vi "Main Page.vi"(8 "error in (no error)":errorcluster, 11 "Node Ptr":T2 format="%.0x") -> (0 "error out":errorcluster)   [LabVIEW 2016, in "DCM System Explorer.lvlib"]
uses:
  DCM System Explorer.lvlib
  <vilib>/NI Veristand/Custom Device API/Custom Device Item Ref.ctl
  Types/Bitfile Selection.ctl
  System.Windows.Forms
  <vilib>/NI Veristand/Custom Device API/Dependent File Optional Info.ctl
  <vilib>/Powertrain Controls/Device Drivers/DCM/Rev0/RT/DCM - RT.lvclass/DCM - RT.ctl
  <vilib>/Powertrain Controls/Device Drivers/DCM/Rev0/RT/Read System.vi
  <vilib>/Powertrain Controls/Device Drivers/DCM/Rev0/RT/Read PB.vi
  Shared/DCM Properties.vi
  <vilib>/NI Veristand/Custom Device API/Set Item Property (Boolean).vi
  Shared/DCM Constants and GUIDs.vi
  <vilib>/NI Veristand/Custom Device API/Get Item Property (String).vi
  <vilib>/NI Veristand/Custom Device API/Get Item Property (I32).vi
  <vilib>/NI Veristand/Custom Device API/Get Item Property (Dependent File).vi
  <vilib>/NI Veristand/Custom Device API/Get Item Property (U16).vi
  SubVIs/Custom Device Ref.vi
  <vilib>/NI Veristand/Custom Device API/Set Item Property (String).vi
  <vilib>/NI Veristand/Custom Device API/Set Item Property (U16).vi
  <vilib>/NI Veristand/Custom Device API/Set Item Property (I32).vi
  <vilib>/NI Veristand/Custom Device API/Set Item Property (Dependent File).vi
  <vilib>/NI Veristand/Custom Device API/Set Item Property (Path).vi
  <vilib>/FPGAPlugInAG/sbRIO-9651/niLvFpga_Open_sbRIO-9651.vi
  <vilib>/rvi/interface/common/dynamic/niFpgaDynamicAddResources.vi
  <vilib>/rvi/interface/nirviOpenFPGA/nirviOpenFPGA.xnode
  <vilib>/Powertrain Controls/Device Drivers/DCM/Top Level/FPGA Bitfiles/DCM - FPGA - Calibration.lvbitx
  <vilib>/NI VeriStand/Custom Device API/Custom Device API.lvlib
  DCM Shared.lvlib
  <vilib>/Powertrain Controls/Device Drivers/DCM/Rev0/RT/DCM - RT.lvclass
panel:
  in  "Password":string
  in  "Username":string
  out "Status":string
  in  "Clear":bool
  in  "Discover":bool
  in  "Header 4":cluster{"Section Name":string}={"Section Name"="Timed Loop Setup"}
  in  "Device Name":string
  in  "CPU-Sys":i32=-2 caption="CPU"
  in  "Rate-Sys":i32=1 caption="Rate decimation" min=1
  in  "Priority-Sys":enum16{"Low", "Medium", "High"}(ring)=enum."Medium" caption="Execution priority"
  in  "CPU-Cmd":i32=-2 caption="CPU"
  in  "Rate-Cmd":i32=1 caption="Rate decimation" min=1
  in  "Priority-Cmd":enum16{"Low", "Medium", "High"}(ring)=enum."Medium" caption="Execution priority"
  in  "Header 3":cluster{"Section Name":string}={"Section Name"="DCM Model & Bitfile Initialization"}
  in  "Header 2":cluster{"Section Name":string}={"Section Name"="FPGA Target Setup"}
  in  "FPGA Resource":string="RIO0"
  in  "IP Address":string
  in  "FPGA Location":enum16{"Local", "Remote"}(ring)
  out "RT File Path":string caption="RT File Path - FPGA Bitfile"
  out "Local File Path":path caption="Local File Path - FPGA Bitfile"
  out "DCM Model":T1
  out "Device Address":string="RIO0"
  out "CD Version":string caption="Custom Device Version"
  in  "Header":cluster{"Section Name":string}={"Section Name"="Real-Time Target Setup"}
  # "Command Loop"
  # "(-2: automatic)"
  # "System Loop"
  # "(-2: automatic)"
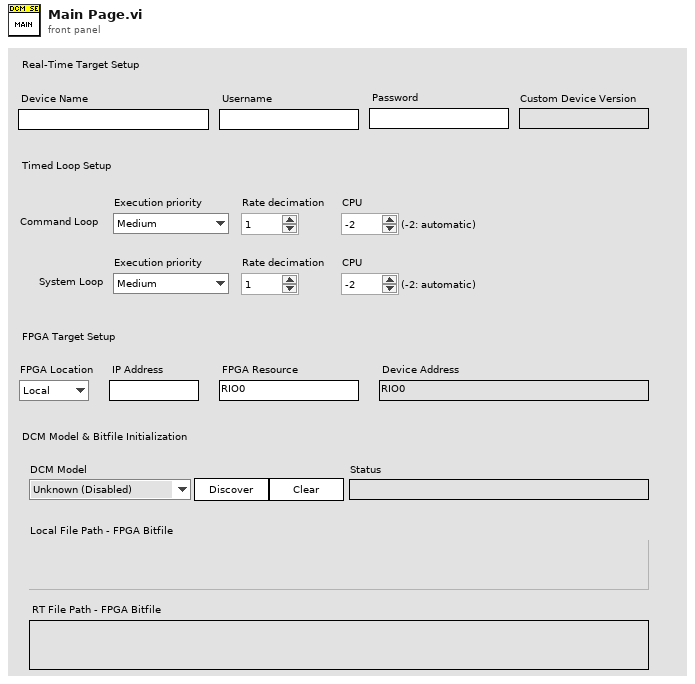
[diagram p1: front panel]
types:
  T1 = typedef "DCM System Explorer.lvlib/Bitfile Selection.ctl" = enum16{"Unknown (Disabled)", "DCM-2301", "DCM-2302", "DCM-2316", "DCM-2317"}
  T2 = typedef "Custom Device API.lvlib/Custom Device Item Ref.ctl" = u64
  T3 = enum8{"Enabled", "Disabled", "Disabled and Grayed Out"}
  T4 = typedef "Custom Device API.lvlib/Dependent File Optional Info.ctl" = cluster{"Version":string, "RTDestination":path, "ForceDownload":bool, "SupportedTarget":string, "MD5":string}
  T5 = typedef "Custom Device API.lvlib/Custom Device Item Info.ctl" = cluster{"Name":string, "Is Channel":bool, "GUID":string, "Is Waveform":bool}
  T6 = typedef "Custom Device API.lvlib/Custom Device Commands.ctl" = enum16{"Default", "Item renamed", "Shutdown", "Dynamic button pressed"}
  T7 = typedef "nirio_resource_slv.ctl" = tag
  T8 = typedef "DCM - RT.lvclass/System.ctl" = cluster{"Model":u16, "Rev Major":u8, "Rev Minor":u8, "Serial Number":u32}
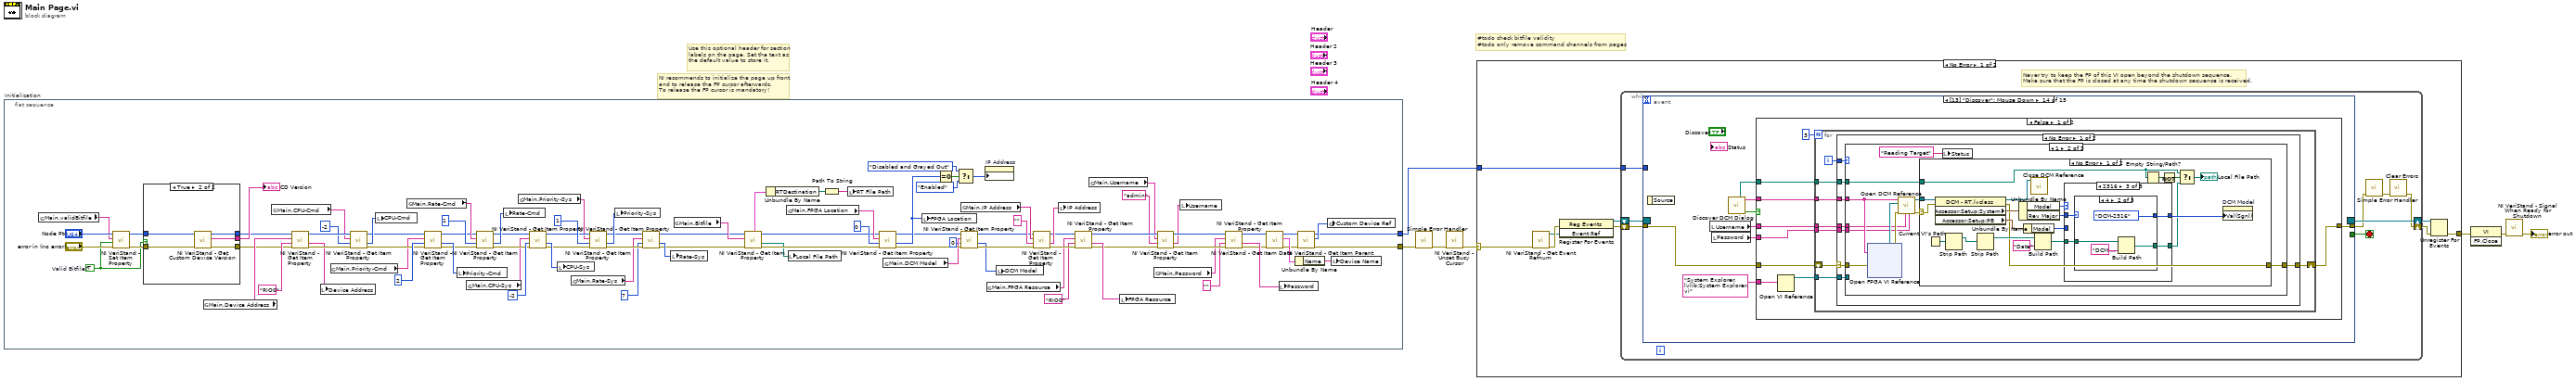
[diagram p0: block diagram]
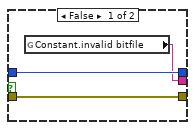
[diagram p2: hidden frame]
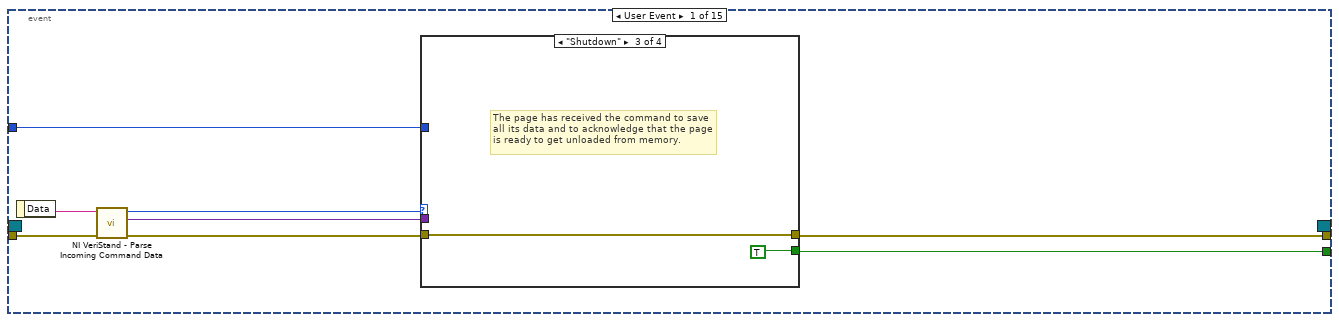
[diagram p3: hidden frame]
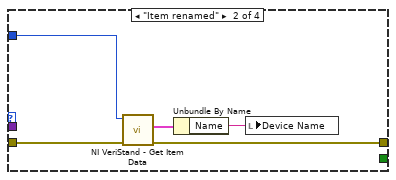
[diagram p5: hidden frame]
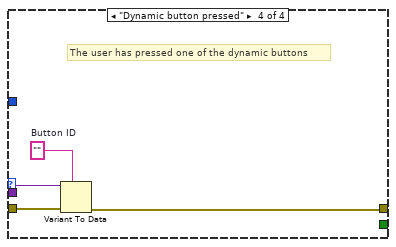
[diagram p6: hidden frame]
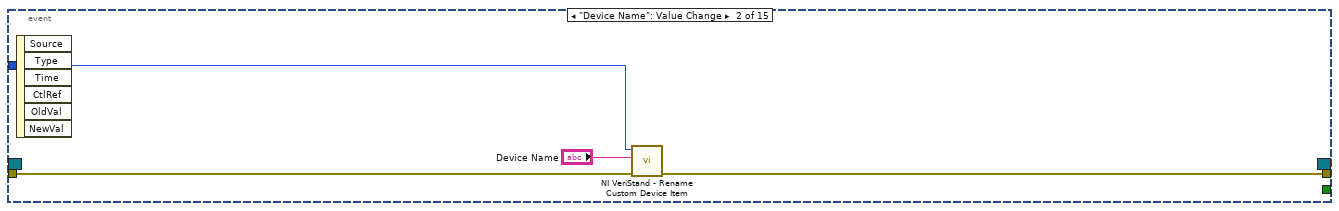
[diagram p7: hidden frame]
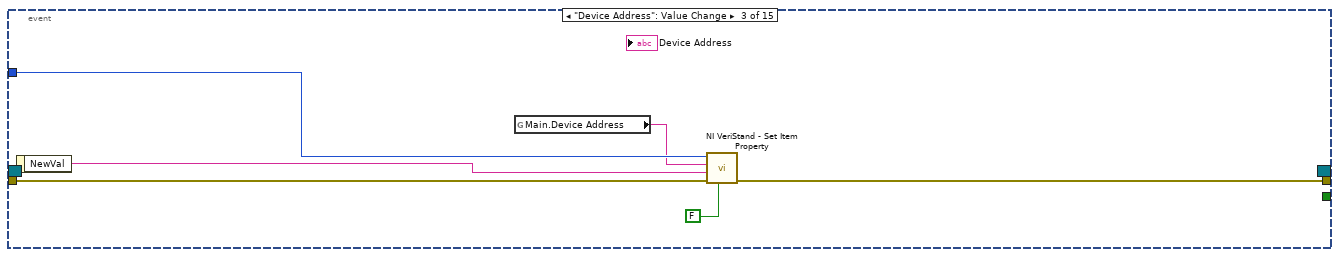
[diagram p8: hidden frame]
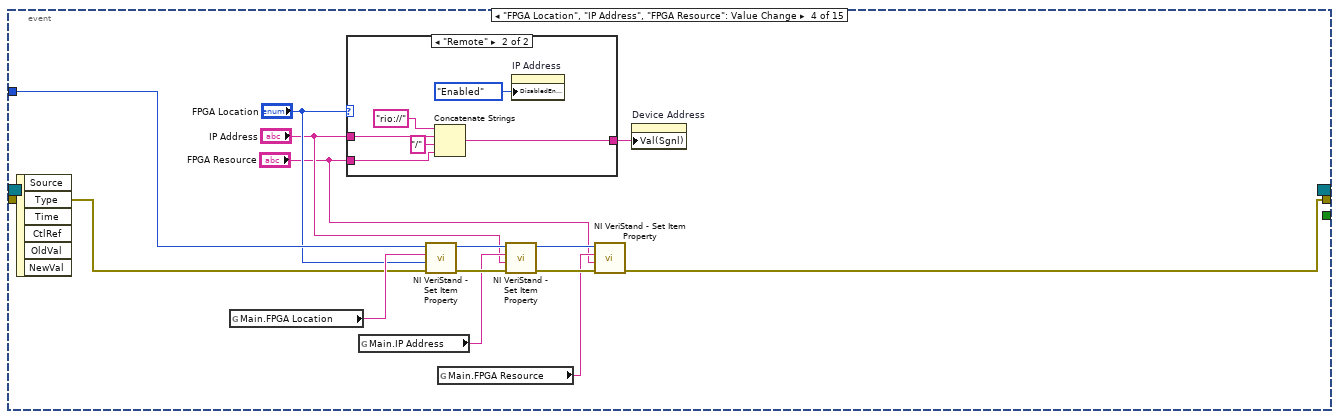
[diagram p9: hidden frame]
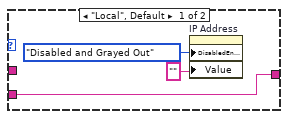
[diagram p10: hidden frame]
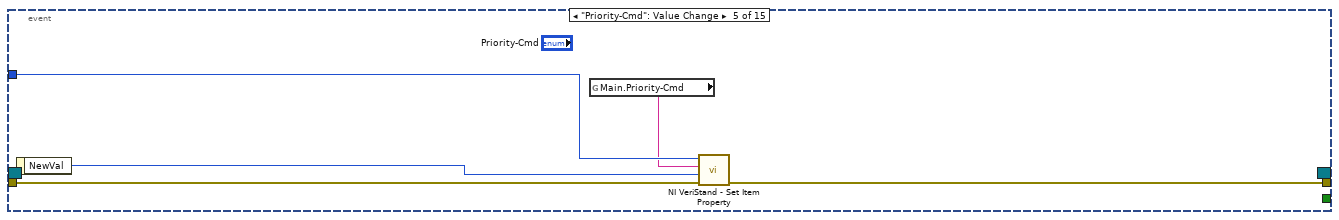
[diagram p11: hidden frame]
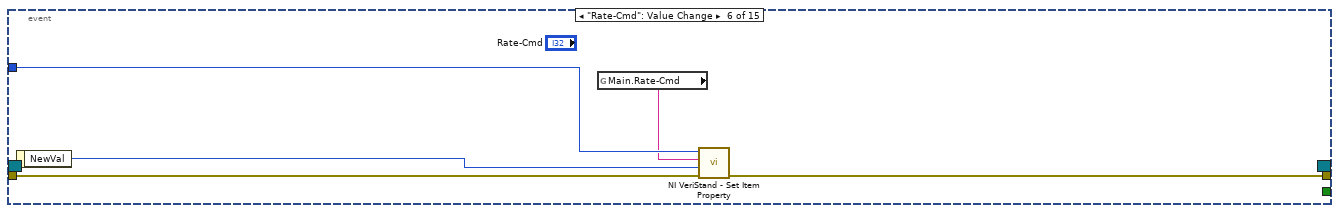
[diagram p12: hidden frame]
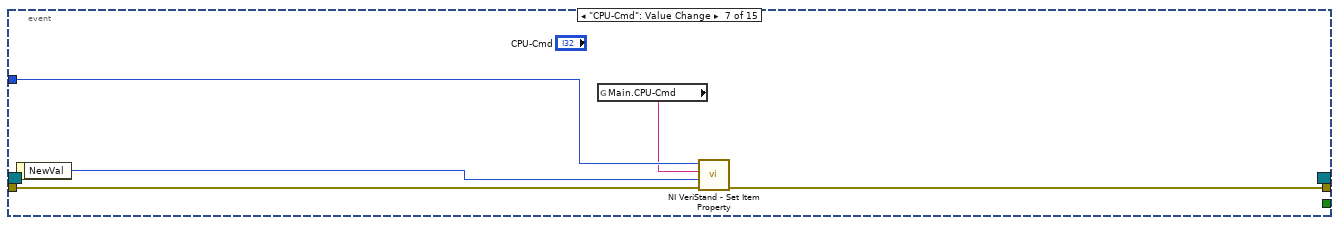
[diagram p13: hidden frame]
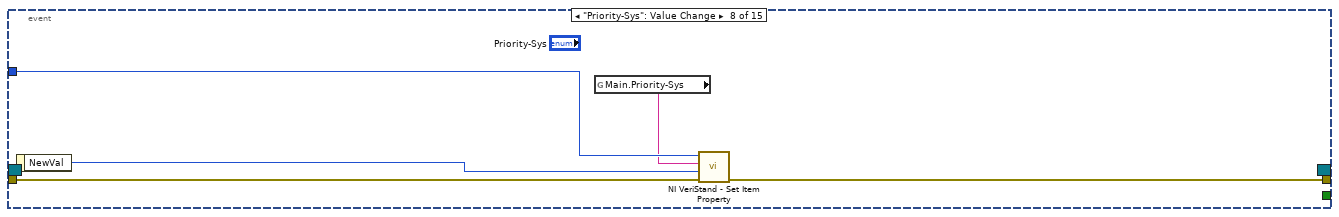
[diagram p14: hidden frame]
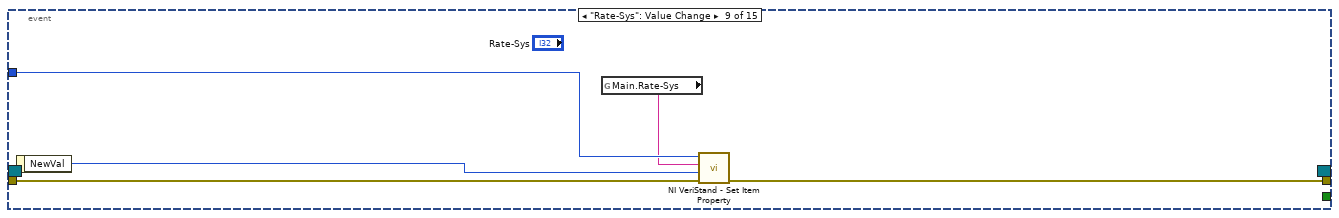
[diagram p15: hidden frame]
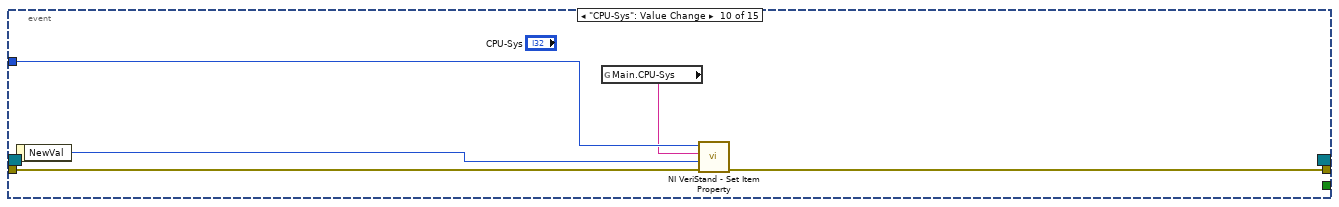
[diagram p16: hidden frame]
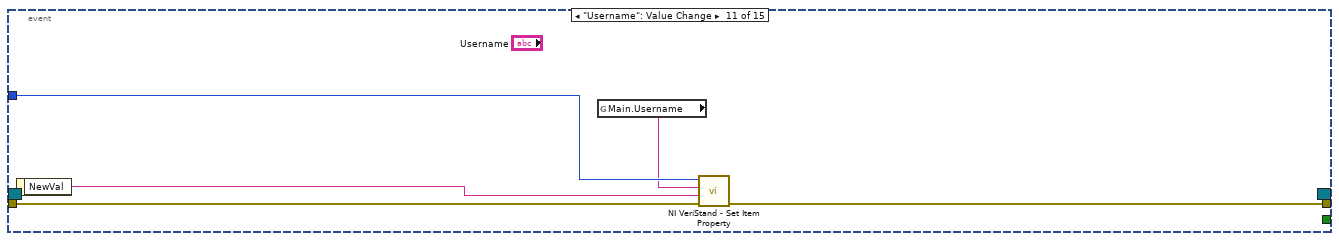
[diagram p17: hidden frame]
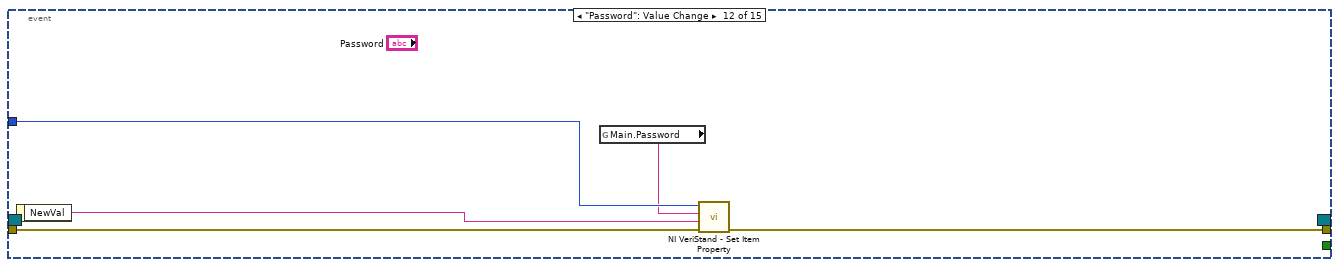
[diagram p18: hidden frame]
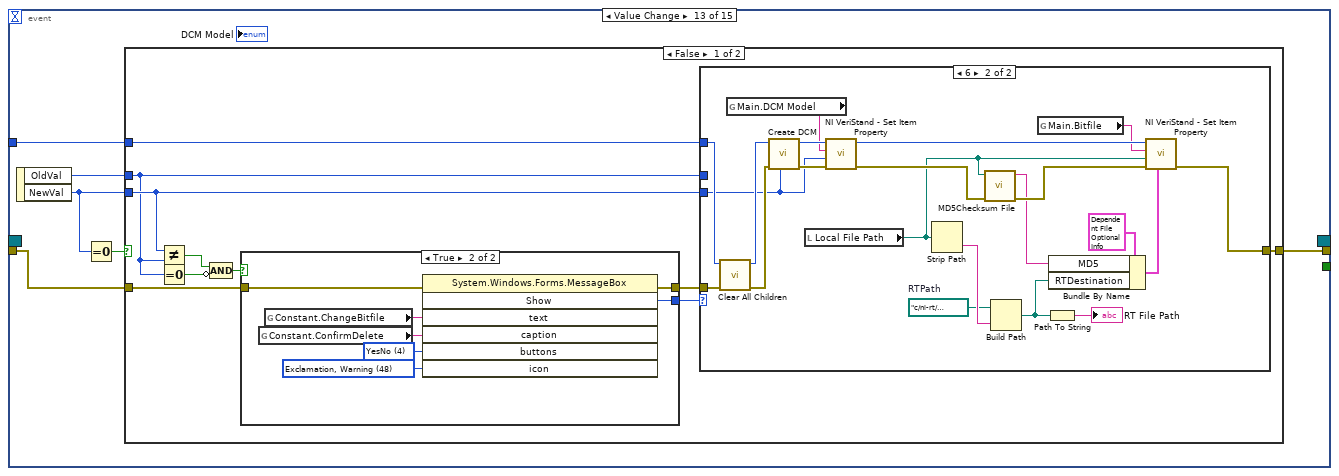
[diagram p19: hidden frame]
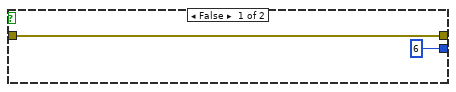
[diagram p20: hidden frame]
diagram:
  # "#todo check bitfile validity\n#todo only remove command channels from pages"
  # "Use this optional header for section labels on the page. Set the text as the default value to store it."
  # "NI recommends to initialize the page up front\nand to release the FP cursor afterwards.\nTo release the FP cursor is mandatory!"
  n1 = flat-sequence "Initialization" {
    tunnel: [w10] -> w3
    tunnel: [w14] -> w2
    frame #0 {
      w84 = TRUE  # Valid Bitfile?
      n2 = global read "DCM Properties.vi" "Main.validBitfile"() -> (w90:string)
      n3 = call-poly <vilib>:"NI VeriStand - Set Item Property.vi"("error in (no error)"="error in (no error)", "Value"=w84, "Property Name"=w90, "Item Ref in"="Node Ptr") -> ("error out"=w88:errorcluster, "Item Ref out"=w89:T2)  [unwired: 5 in, 1 out]
      n4 = case shown="True" w84 {
        tunnel: [w101 w107] -> w61
        tunnel: [w102 w106] -> w62
        tunnel: w89 -> [w102 w105]
        tunnel: w88 -> [w101 w104]
        tunnel: [w100 w103] -> w87
        frame False {
          n5 = global read "DCM Constants and GUIDs.vi" "Constant.invalid bitfile"() -> (w100:string)
        }
        frame True {
          n6 = call <vilib>:"NI VeriStand - Get Custom Device Version.vi"("error in (no error)"=w104, "Device Ref in"=w105) -> ("error out"=w107:errorcluster, "Value"=w103:string, "Device Ref out"=w106:T2)  [unwired: 7 in]
        }
      }
      "CD Version" <- w87
      n7 = global read "DCM Properties.vi" "Main.Device Address"() -> (w86:string)
      n8 = global read "DCM Properties.vi" "Main.CPU-Cmd"() -> (w85:string)
      n9 = call-poly <vilib>:"NI VeriStand - Get Item Property.vi"("error in (no error)"=w61, "Default Value"="RIO0", "Property Name"=w86, "Item Ref in"=w62) -> ("error out"=w96:errorcluster, "Value"=w83:string, "Item Ref out"=w93:T2)  [unwired: 4 in, 1 out]
      n10 = local write "Device Address"(w83) -> ()
      n11 = global read "DCM Properties.vi" "Main.Priority-Cmd"() -> (w60:string)
      n12 = call-poly <vilib>:"NI VeriStand - Get Item Property.vi"("error in (no error)"=w96, "Default Value"=-2, "Property Name"=w85, "Item Ref in"=w93) -> ("error out"=w65:errorcluster, "Value"=w91:i32, "Item Ref out"=w66:T2)  [unwired: 4 in, 1 out]
      n13 = local write "CPU-Cmd"(w91) -> ()
      n14 = global read "DCM Properties.vi" "Main.Rate-Cmd"() -> (w59:string)
      n15 = call-poly <vilib>:"NI VeriStand - Get Item Property.vi"("error in (no error)"=w65, "Default Value"=2, "Property Name"=w60, "Item Ref in"=w66) -> ("error out"=w64:errorcluster, "Value"=w72:i32, "Item Ref out"=w56:T2)  [unwired: 4 in, 1 out]
      n16 = local write "Priority-Cmd"(w72) -> ()
      n17 = global read "DCM Properties.vi" "Main.CPU-Sys"() -> (w58:string)
      n18 = call-poly <vilib>:"NI VeriStand - Get Item Property.vi"("error in (no error)"=w64, "Default Value"=1, "Property Name"=w59, "Item Ref in"=w56) -> ("error out"=w63:errorcluster, "Value"=w69:i32, "Item Ref out"=w57:T2)  [unwired: 4 in, 1 out]
      n19 = local write "Rate-Cmd"(w69) -> ()
      n20 = global read "DCM Properties.vi" "Main.Priority-Sys"() -> (w46:string)
      n21 = call-poly <vilib>:"NI VeriStand - Get Item Property.vi"("error in (no error)"=w63, "Default Value"=-2, "Property Name"=w58, "Item Ref in"=w57) -> ("error out"=w49:errorcluster, "Value"=w68:i32, "Item Ref out"=w52:T2)  [unwired: 4 in, 1 out]
      n22 = local write "CPU-Sys"(w68) -> ()
      n23 = global read "DCM Properties.vi" "Main.Rate-Sys"() -> (w48:string)
      n24 = call-poly <vilib>:"NI VeriStand - Get Item Property.vi"("error in (no error)"=w49, "Default Value"=1, "Property Name"=w46, "Item Ref in"=w52) -> ("error out"=w50:errorcluster, "Value"=w54:i32, "Item Ref out"=w51:T2)  [unwired: 4 in, 1 out]
      n25 = local write "Priority-Sys"(w54) -> ()
      n26 = call-poly <vilib>:"NI VeriStand - Get Item Property.vi"("error in (no error)"=w50, "Default Value"=7, "Property Name"=w48, "Item Ref in"=w51) -> ("error out"=w27:errorcluster, "Value"=w55:i32, "Item Ref out"=w26:T2)  [unwired: 4 in, 1 out]
      n27 = local write "Rate-Sys"(w55) -> ()
      n28 = global read "DCM Properties.vi" "Main.Bitfile"() -> (w31:string)
      n29 = call-poly <vilib>:"NI VeriStand - Get Item Property.vi"("error in (no error)"=w27, "Property Name"=w31, "Item Ref in"=w26) -> ("error out"=w32:errorcluster, "Path"=w25:path, "Item Ref out"=w33:T2, "OptionalInfo"=w30:T4)  [unwired: 4 in, 1 out]
      n30 = Unbundle By Name(w30) -> ("RTDestination"=w29:path)
      n31 = global read "DCM Properties.vi" "Main.FPGA Location"() -> (w81:string)
      n32 = local write "Local File Path"(w25) -> ()
      n33 = Path To String(path=w29) -> (string=w28:string)
      n34 = local write "RT File Path"(w28) -> ()
      n35 = call-poly <vilib>:"NI VeriStand - Get Item Property.vi"("error in (no error)"=w32, "Default Value"=u16 0, "Property Name"=w81, "Item Ref in"=w33) -> ("error out"=w39:errorcluster, "Value"=w41:u16, "Item Ref out"=w40:T2)  [unwired: 4 in, 1 out]
      n36 = global read "DCM Properties.vi" "Main.DCM Model"() -> (w36:string)
      n37 = local write "FPGA Location"(w41) -> ()
      n38 = Equal To 0?(x=w41) -> (x = 0?=w42:bool)
      n39 = Select(t=T3."Disabled and Grayed Out" ("Disabled"), s=w42, f=T3."Enabled" ("Disabled")) -> (s? t:f=w43:T3)
      n40 = global read "DCM Properties.vi" "Main.IP Address"() -> (w80:string)
      n41 = call-poly <vilib>:"NI VeriStand - Get Item Property.vi"("error in (no error)"=w39, "Default Value"=u16 0, "Property Name"=w36, "Item Ref in"=w40) -> ("error out"=w38:errorcluster, "Value"=w34:u16, "Item Ref out"=w37:T2)  [unwired: 4 in, 1 out]
      n42 = property on="IP Address" class="Str"("DisabledEnum"=w43) -> ()  [unwired: 2 in, 2 out]
      n43 = global read "DCM Properties.vi" "Main.FPGA Resource"() -> (w74:string)
      n44 = local write "DCM Model"(w34) -> ()
      n45 = call-poly <vilib>:"NI VeriStand - Get Item Property.vi"("error in (no error)"=w38, "Default Value"="", "Property Name"=w80, "Item Ref in"=w37) -> ("error out"=w76:errorcluster, "Value"=w78:string, "Item Ref out"=w77:T2)  [unwired: 4 in, 1 out]
      n46 = local write "IP Address"(w78) -> ()
      n47 = call-poly <vilib>:"NI VeriStand - Get Item Property.vi"("error in (no error)"=w76, "Default Value"="RIO0", "Property Name"=w74, "Item Ref in"=w77) -> ("error out"=w23:errorcluster, "Value"=w75:string, "Item Ref out"=w24:T2)  [unwired: 4 in, 1 out]
      n48 = global read "DCM Properties.vi" "Main.Username"() -> (w20:string)
      n49 = local write "FPGA Resource"(w75) -> ()
      n50 = global read "DCM Properties.vi" "Main.Password"() -> (w17:string)
      n51 = call-poly <vilib>:"NI VeriStand - Get Item Property.vi"("error in (no error)"=w23, "Default Value"="admin", "Property Name"=w20, "Item Ref in"=w24) -> ("error out"=w21:errorcluster, "Value"=w18:string, "Item Ref out"=w22:T2)  [unwired: 4 in, 1 out]
      n52 = local write "Username"(w18) -> ()
      n53 = call-poly <vilib>:"NI VeriStand - Get Item Property.vi"("error in (no error)"=w21, "Default Value"="", "Property Name"=w17, "Item Ref in"=w22) -> ("error out"=w8:errorcluster, "Value"=w15:string, "Item Ref out"=w9:T2)  [unwired: 4 in, 1 out]
      n54 = call <vilib>:"NI VeriStand - Get Item Data.vi"("error in (no error)"=w8, "Item Ref in"=w9) -> ("error out"=w13:errorcluster, "Item Info"=w98:T5, "Item Ref out"=w12:T2)  [unwired: 7 out]
      n55 = local write "Password"(w15) -> ()
      n56 = Unbundle By Name(w98) -> ("Name"=w97:string)
      n57 = call <vilib>:"NI VeriStand - Get Item Parent.vi"("error in (no error)"=w13, "Item Ref in"=w12) -> ("error out"=w14:errorcluster, "Parent Ref"=w11:T2, "Item Ref out"=w10:T2)  [unwired: 6 in, 1 out]
      n58 = global write "Custom Device Ref.vi" "Custom Device Ref"(w11) -> ()
      n59 = local write "Device Name"(w97) -> ()
    }
  }
  n60 = call <vilib>:"Simple Error Handler.vi"("error in (no error)"=w2) -> ("error out"=w1:errorcluster)  [unwired: 1 in, 7 out]
  n61 = call <vilib>:"NI VeriStand - Unset Busy Cursor.vi"("error in (no error)"=w1) -> ("error out"=w4:errorcluster)  [unwired: 10 out]
  n62 = case shown="No Error" w4 {
    selector: w4 -> [w109 w403]
    tunnel: [w113 w401] -> w7
    tunnel: w3 -> [w108 _]
    frame No Error {
      # "Never try to keep the FP of this VI open beyond the shutdown sequence.\nMake sure that the FP is closed at any time the shutdown sequence is received."
      n63 = call <vilib>:"NI VeriStand - Get Event Refnum.vi"("error in (no error)"=w109) -> ("error out"=w116:errorcluster, "Event Ref"=w112:refnum<user-event>)  [unwired: 9 out]
      n64 = register-events(error in=w116, w112) -> (reference out=w110:refnum<event-registration>, error out=w111:errorcluster)  [unwired: 1 in]
      n65 = while {
        shift-right: [w118] -> w114
        shift-left: w111 -> [w123]
        shift-right: [w124] -> w115
        shift-left: w110 -> [w122]
        tunnel: w108 -> [w117]
        stop <- w121 stop-if-true
        n66 = event shown="[13] \"Discover\": Mouse Down" {
          selector: w122 -> [_ _ _ _ _ _ _ _ _ _ _ _ _ _ _]
          dyn-events: [_ _ _ _ _ _ _ _ _ _ _ _ _ _ _] -> w124
          timeout: _ -> [_ _ _ _ _ _ _ _ _ _ _ _ _ _ _]
          tunnel: w123 -> [w132 w148 w154 w160 w182 w187 w192 w197 w202 w207 w212 w217 w223 w302 _]
          tunnel: [w128 _ _ _ _ _ _ _ _ _ _ _ _ _ _] -> w121
          tunnel: [w127 w147 w152 w159 w180 w185 w190 w195 w200 w205 w210 w215 w222 w301 _] -> w120
          tunnel: w117 -> [w125 w146 w150 w166 w179 w184 w189 w194 w199 w204 w209 w214 w221 _ _]
          event User Event {
            n67 = event-data() -> ("Data"=w131:string)  [unwired: 1 out]
            n68 = call <vilib>:"NI VeriStand - Parse Incoming Command Data.vi"("error in (no error)"=w132, "Incoming data"=w131) -> ("error out"=w130:errorcluster, "Outgoing data"=w126:variant, "Action"=w129:T6)  [unwired: 7 out]
            n69 = case shown="\"Shutdown\"" w129 {
              tunnel: w130 -> [w133 w138 w139 w144]
              tunnel: [_ _ TRUE _] -> w128
              tunnel: [w133 w136 w139 w141] -> w127
              tunnel: w126 -> [_ _ _ w143]
              tunnel: w125 -> [_ w134 _ _]
              frame "Default", Default {
              }
              frame "Item renamed" {
                n70 = call <vilib>:"NI VeriStand - Get Item Data.vi"("error in (no error)"=w138, "Item Ref in"=w134) -> ("error out"=w136:errorcluster, "Item Info"=w137:T5)  [unwired: 8 out]
                n71 = Unbundle By Name(w137) -> ("Name"=w135:string)
                n72 = local write "Device Name"(w135) -> ()
              }
              frame "Shutdown" {
                # "The page has received the command to save all its data and to acknowledge that the page is ready to get unloaded from memory."
              }
              frame "Dynamic button pressed" {
                w142 = ""  # Button ID
                # "The user has pressed one of the dynamic buttons"
                n73 = Variant To Data(error in=w144, type=w142, Variant=w143) -> (error out=w141:errorcluster)  [unwired: 1 out]
              }
            }
          }
          event "Device Name": Value Change {
            n74 = event-data() -> ()  [unwired: 7 out]
            n75 = call <vilib>:"NI VeriStand - Rename Custom Device Item.vi"("error in (no error)"=w148, "New Name"="Device Name", "Item Ref in"=w146) -> ("error out"=w147:errorcluster)  [unwired: 1 in, 7 out]
          }
          event "Device Address": Value Change {
            n76 = event-data() -> ("NewVal"=w153:string)  [unwired: 1 out]
            n77 = global read "DCM Properties.vi" "Main.Device Address"() -> (w149:string)
            n78 = call-poly <vilib>:"NI VeriStand - Set Item Property.vi"("Binary String (T)"=FALSE, "error in (no error)"=w154, "Value"=w153, "Property Name"=w149, "Item Ref in"=w150) -> ("error out"=w152:errorcluster)  [unwired: 4 in, 2 out]
          }
          event "FPGA Location", "IP Address", "FPGA Resource": Value Change {
            n79 = event-data() -> ()  [unwired: 7 out]
            n80 = global read "DCM Properties.vi" "Main.FPGA Location"() -> (w167:string)
            n81 = case shown="\"Remote\"" "FPGA Location" {
              tunnel: "IP Address" -> [_ w176]
              tunnel: "FPGA Resource" -> [w171 w175]
              tunnel: [w171 w173] -> w168
              frame "Local", Default {
                n82 = property on="IP Address" class="Str"("DisabledEnum"=T3."Disabled and Grayed Out" ("Disabled"), "Value"="" ("IP Address")) -> ()  [unwired: 2 in, 2 out]
              }
              frame "Remote" {
                n83 = Concatenate Strings("rio://", w176, "/" ("string"), w175) -> (w173:string)
                n84 = property on="IP Address" class="Str"("DisabledEnum"=T3."Enabled" ("Disabled")) -> ()  [unwired: 2 in, 2 out]
              }
            }
            n85 = global read "DCM Properties.vi" "Main.IP Address"() -> (w157:string)
            n86 = call-poly <vilib>:"NI VeriStand - Set Item Property.vi"("error in (no error)"=w160, "Value"="FPGA Location", "Property Name"=w167, "Item Ref in"=w166) -> ("error out"=w163:errorcluster, "Item Ref out"=w164:T2)  [unwired: 5 in, 1 out]
            n87 = global read "DCM Properties.vi" "Main.FPGA Resource"() -> (w158:string)
            n88 = call-poly <vilib>:"NI VeriStand - Set Item Property.vi"("error in (no error)"=w163, "Value"="IP Address", "Property Name"=w157, "Item Ref in"=w164) -> ("error out"=w162:errorcluster, "Item Ref out"=w161:T2)  [unwired: 5 in, 1 out]
            n89 = call-poly <vilib>:"NI VeriStand - Set Item Property.vi"("error in (no error)"=w162, "Value"="FPGA Resource", "Property Name"=w158, "Item Ref in"=w161) -> ("error out"=w159:errorcluster)  [unwired: 5 in, 2 out]
            n90 = property on="Device Address" class="Str"("Val(Sgnl)"=w168) -> ()  [unwired: 2 in, 2 out]
          }
          event "Priority-Cmd": Value Change {
            n91 = event-data() -> ("NewVal"=w181:enum16{"Low", "Medium", "High"})  [unwired: 1 out]
            n92 = global read "DCM Properties.vi" "Main.Priority-Cmd"() -> (w178:string)
            n93 = call-poly <vilib>:"NI VeriStand - Set Item Property.vi"("error in (no error)"=w182, "Value"=w181, "Property Name"=w178, "Item Ref in"=w179) -> ("error out"=w180:errorcluster)  [unwired: 5 in, 2 out]
          }
          event "Rate-Cmd": Value Change {
            n94 = event-data() -> ("NewVal"=w186:i32)  [unwired: 1 out]
            n95 = global read "DCM Properties.vi" "Main.Rate-Cmd"() -> (w183:string)
            n96 = call-poly <vilib>:"NI VeriStand - Set Item Property.vi"("error in (no error)"=w187, "Value"=w186, "Property Name"=w183, "Item Ref in"=w184) -> ("error out"=w185:errorcluster)  [unwired: 5 in, 2 out]
          }
          event "CPU-Cmd": Value Change {
            n97 = event-data() -> ("NewVal"=w191:i32)  [unwired: 1 out]
            n98 = global read "DCM Properties.vi" "Main.CPU-Cmd"() -> (w188:string)
            n99 = call-poly <vilib>:"NI VeriStand - Set Item Property.vi"("error in (no error)"=w192, "Value"=w191, "Property Name"=w188, "Item Ref in"=w189) -> ("error out"=w190:errorcluster)  [unwired: 5 in, 2 out]
          }
          event "Priority-Sys": Value Change {
            n100 = event-data() -> ("NewVal"=w196:enum16{"Low", "Medium", "High"})  [unwired: 1 out]
            n101 = global read "DCM Properties.vi" "Main.Priority-Sys"() -> (w193:string)
            n102 = call-poly <vilib>:"NI VeriStand - Set Item Property.vi"("error in (no error)"=w197, "Value"=w196, "Property Name"=w193, "Item Ref in"=w194) -> ("error out"=w195:errorcluster)  [unwired: 5 in, 2 out]
          }
          event "Rate-Sys": Value Change {
            n103 = event-data() -> ("NewVal"=w201:i32)  [unwired: 1 out]
            n104 = global read "DCM Properties.vi" "Main.Rate-Sys"() -> (w198:string)
            n105 = call-poly <vilib>:"NI VeriStand - Set Item Property.vi"("error in (no error)"=w202, "Value"=w201, "Property Name"=w198, "Item Ref in"=w199) -> ("error out"=w200:errorcluster)  [unwired: 5 in, 2 out]
          }
          event "CPU-Sys": Value Change {
            n106 = event-data() -> ("NewVal"=w206:i32)  [unwired: 1 out]
            n107 = global read "DCM Properties.vi" "Main.CPU-Sys"() -> (w203:string)
            n108 = call-poly <vilib>:"NI VeriStand - Set Item Property.vi"("error in (no error)"=w207, "Value"=w206, "Property Name"=w203, "Item Ref in"=w204) -> ("error out"=w205:errorcluster)  [unwired: 5 in, 2 out]
          }
          event "Username": Value Change {
            n109 = event-data() -> ("NewVal"=w211:string)  [unwired: 1 out]
            n110 = global read "DCM Properties.vi" "Main.Username"() -> (w208:string)
            n111 = call-poly <vilib>:"NI VeriStand - Set Item Property.vi"("error in (no error)"=w212, "Value"=w211, "Property Name"=w208, "Item Ref in"=w209) -> ("error out"=w210:errorcluster)  [unwired: 5 in, 2 out]
          }
          event "Password": Value Change {
            n112 = event-data() -> ("NewVal"=w216:string)  [unwired: 1 out]
            n113 = global read "DCM Properties.vi" "Main.Password"() -> (w213:string)
            n114 = call-poly <vilib>:"NI VeriStand - Set Item Property.vi"("error in (no error)"=w217, "Value"=w216, "Property Name"=w213, "Item Ref in"=w214) -> ("error out"=w215:errorcluster)  [unwired: 5 in, 2 out]
          }
          event Value Change {
            n115 = event-data() -> ("OldVal"=w218:T1, "NewVal"=w219:T1)  [unwired: 1 out]
            n116 = Equal To 0?(x=w219) -> (x = 0?=w220:bool)
            n117 = case shown="False" w220 {
              tunnel: w223 -> [w233 w272]
              tunnel: [w232 w268] -> w222
              tunnel: w221 -> [w224 w267]
              tunnel: w219 -> [w226 w266]
              tunnel: w218 -> [w225 w270]
              frame False {
                n118 = Not Equal?(x=w226, y=w225) -> (x != y?=w227:bool)
                n119 = Equal To 0?(x=w225) -> (x = 0?=w229:bool)
                n120 = Compound Arithmetic op=AND(w227, invert w229) -> (w228:bool)
                n121 = case shown="True" w228 {
                  tunnel: w233 -> [w235 w240]
                  tunnel: [6 ("Show") w239] -> w231
                  tunnel: [w235 w238] -> w230
                  frame False {
                  }
                  frame True {
                    w242 = 4 items=["OK", "OKCancel", "AbortRetryIgnore", "YesNoCancel", "YesNo", "RetryCancel"] ("buttons")
                    w241 = 48 items=["None"=0, "Hand, Error, Stop"=16, "Question"=32, "Exclamation, Warning"=48, "Asterisk, Information"=64] ("icon")
                    n122 = global read "DCM Constants and GUIDs.vi" "Constant.ConfirmDelete"() -> (w236:string)
                    n123 = global read "DCM Constants and GUIDs.vi" "Constant.ChangeBitfile"() -> (w237:string)
                    n124 = invoke class="System.Windows.Forms.MessageBox" method="Show"(error in=w240, "text"=w237, "caption"=w236, "buttons"=w242, "icon"=w241) -> (error out=w238:errorcluster, "Show"=w239:i32)  [unwired: 2 in, 5 out]
                  }
                }
                n125 = case shown="6" w231 {
                  tunnel: w230 -> [w244 w265]
                  tunnel: [w244 w245] -> w232
                  tunnel: w224 -> [_ w263]
                  tunnel: w226 -> [_ w256]
                  tunnel: w225 -> [w243 _]
                  frame 7, Default {
                    n126 = local write "DCM Model"(w243) -> ()
                  }
                  frame 6 {
                    w249 = path "c:/ni-rt/NIVeriStand/Custom Devices/DCM"  # RTPath
                    n127 = call "Clear All Children.vi"("error in (no error)"=w265, "Item Ref in"=w263) -> ("error out"=w264:errorcluster, "Item Ref out"=w262:T2)  [unwired: 8 in]
                    n128 = global read "DCM Properties.vi" "Main.DCM Model"() -> (w257:string)
                    n129 = call "Create DCM.vi"("DCM Model"=w256, "error in (no error)"=w264, "Section Ptr"=w262) -> ("error out"=w260:errorcluster, "Section Ptr dup"=w261:T2)  [unwired: 7 in]
                    n130 = local read "Local File Path"() -> (w246:path)
                    n131 = call-poly <vilib>:"NI VeriStand - Set Item Property.vi"("error in (no error)"=w260, "Value"=w256, "Property Name"=w257, "Item Ref in"=w261) -> ("error out"=w259:errorcluster, "Item Ref out"=w258:T2)  [unwired: 5 in, 1 out]
                    n132 = Strip Path(path=w246) -> (name=w250:string)  [unwired: 1 out]
                    n133 = call <vilib>:"MD5Checksum File.vi"("error in (no error)"=w259, "Path"=w246) -> ("error out"=w252:errorcluster, "MD5 message-digest"=w248:string)  [unwired: 8 in]
                    n134 = Build Path(base path=w249, name or relative path=w250) -> (appended path=w247:path)
                    n135 = global read "DCM Properties.vi" "Main.Bitfile"() -> (w255:string)
                    n136 = Path To String(path=w247) -> (string=→"RT File Path":string)
                    n137 = Bundle By Name(cluster=T4 {"Version"="1.0", "RTDestination"=path "home/lvuser/natinst/NIVeriStand/Custom Devices/DCM-2116", "ForceDownload"=FALSE, "SupportedTarget"="All", "MD5"=""} ("OptionalInfo"), "MD5"=w248, "RTDestination"=w247) -> (w253:T4)
                    n138 = call-poly <vilib>:"NI VeriStand - Set Item Property.vi"("OptionalInfo"=w253, "error in (no error)"=w252, "Path"=w246, "Property Name"=w255, "Item Ref in"=w258) -> ("error out"=w245:errorcluster)  [unwired: 4 in, 2 out]
                  }
                }
              }
              frame True {
                w276 = 4 items=["OK", "OKCancel", "AbortRetryIgnore", "YesNoCancel", "YesNo", "RetryCancel"] ("buttons")
                w275 = 48 items=["None"=0, "Hand, Error, Stop"=16, "Question"=32, "Exclamation, Warning"=48, "Asterisk, Information"=64] ("icon")
                n139 = global read "DCM Constants and GUIDs.vi" "Constant.ConfirmDelete"() -> (w273:string)
                n140 = global read "DCM Constants and GUIDs.vi" "Constant.RemoveBitfile"() -> (w274:string)
                n141 = invoke class="System.Windows.Forms.MessageBox" method="Show"(error in=w272, "text"=w274, "caption"=w273, "buttons"=w276, "icon"=w275) -> (error out=w269:errorcluster, "Show"=w271:i32)  [unwired: 2 in, 5 out]
                n142 = case shown="6" w271 {
                  tunnel: w270 -> [_ w294]
                  tunnel: w269 -> [w289 w293]
                  tunnel: [w292 w293] -> w268
                  tunnel: w267 -> [w290 _]
                  tunnel: w266 -> [w288 _]
                  frame 6 {
                    w278 = path "" ("Value")
                    n143 = global read "DCM Properties.vi" "Main.DCM Model"() -> (w291:string)
                    n144 = call-poly <vilib>:"NI VeriStand - Set Item Property.vi"("error in (no error)"=w289, "Value"=w288, "Property Name"=w291, "Item Ref in"=w290) -> ("error out"=w286:errorcluster, "Item Ref out"=w287:T2)  [unwired: 5 in, 1 out]
                    n145 = local write "RT File Path"("" ("RT File Path")) -> ()
                    n146 = local write "Local File Path"(path "" ("Local File Path")) -> ()
                    n147 = global read "DCM Properties.vi" "Main.Bitfile Path"() -> (w285:string)
                    n148 = call-poly <vilib>:"NI VeriStand - Set Item Property.vi"("error in (no error)"=w286, "Value"=w278, "Property Name"=w285, "Item Ref in"=w287) -> ("error out"=w279:errorcluster, "Item Ref out"=w282:T2)  [unwired: 5 in, 1 out]
                    n149 = global read "DCM Properties.vi" "Main.Bitfile"() -> (w277:string)
                    n150 = call-poly <vilib>:"NI VeriStand - Set Item Property.vi"("error in (no error)"=w279, "Path"=w278, "Property Name"=w277, "Item Ref in"=w282) -> ("error out"=w280:errorcluster, "Item Ref out"=w281:T2)  [unwired: 5 in, 1 out]
                    n151 = call "Clear All Children.vi"("error in (no error)"=w280, "Item Ref in"=w281) -> ("error out"=w292:errorcluster)  [unwired: 8 in, 1 out]
                  }
                  frame 7, Default {
                    n152 = local write "DCM Model"(w294) -> ()
                  }
                }
              }
            }
          }
          event "Discover": Mouse Down {
            n153 = event-data() -> ()  [unwired: 2 out]
            n154 = local read "Username"() -> (w296:string)
            n155 = local read "Password"() -> (w295:string)
            n156 = call "Discover DCM Dialog.vi"() -> ("Canceled?"=w300:bool, "DCM Target Out"=w299:T7, "Path Out"=w297:path)  [unwired: 9 in]
            n157 = case shown="False" w300 {
              tunnel: w302 -> [w311 w399]
              tunnel: [w310 w399] -> w301
              tunnel: w299 -> [w309 _]
              tunnel: "System Explorer.lvlib:System Explorer.vi" ("Status") -> [w306 _]
              tunnel: w297 -> [w305 _]
              tunnel: w296 -> [w304 _]
              tunnel: w295 -> [w303 _]
              frame False {
                n158 = Open VI Reference(vi path=w306) -> (vi reference=w307:refnum<vi>)  [unwired: 5 in, 1 out]
                n159 = for {
                  N: 3 -> [_]
                  shift-right: [w319] -> w310
                  shift-left: w311 -> [w316]
                  tunnel: w309 -> [w317]
                  tunnel: w307 -> [w315]
                  tunnel: w305 -> [w314]
                  tunnel: w304 -> [w313]
                  tunnel: w303 -> [w312]
                  i -> [w318]
                  n160 = case shown="No Error" w316 {
                    selector: w316 -> [w324 w398]
                    tunnel: [w327 w398] -> w319
                    tunnel: w318 -> [w326 _]
                    tunnel: w317 -> [w325 _]
                    tunnel: w315 -> [w323 w396]
                    tunnel: w314 -> [w322 _]
                    tunnel: w313 -> [w321 _]
                    tunnel: w312 -> [w320 _]
                    frame No Error {
                      n161 = case shown="1" w326 {
                        tunnel: [w328 w331 w391] -> w327
                        tunnel: w324 -> [w329 w340 w392]
                        tunnel: w325 -> [_ w337 _]
                        tunnel: w323 -> [w330 _ w394]
                        tunnel: w322 -> [_ w334 _]
                        tunnel: w321 -> [_ w333 _]
                        tunnel: w320 -> [_ w332 _]
                        frame 0 {
                          n162 = call <vilib>:"Set Busy.vi"("error in (no error)"=w329, "VI reference (current VI)"=w330) -> ("error out"=w328:errorcluster)  [unwired: 8 in, 1 out]
                        }
                        frame 1 {
                          n163 = xnode "Open FPGA VI Reference"("error in"=w340, "resource name"=w337) -> ("FPGA VI Reference Out"=w338:refnum<k20>, "error out"=w339:errorcluster)
                          n164 = call <vilib>:"Open DCM Reference.vi"("Password"=w332, "User Name"=w333, "Error In"=w339, "FPGA Reference"=w338, "RIO"=w337) -> ("Error Out"=w335:errorcluster, "DCM Reference"=w336:refnum<class "DCM - RT.lvclass">)  [unwired: 5 in]
                          n165 = case shown="No Error" w335 {
                            selector: w335 -> [w355 w389]
                            tunnel: w336 -> [w356 w390]
                            tunnel: w334 -> [w348 _]
                            tunnel: [w343 w389] -> w331
                            frame No Error {
                              n166 = Current VI's Path() -> (path=w353:path)
                              n167 = property class="DCM - RT.lvclass"(reference=w356, error in=w355) -> (reference out=w354:refnum<class "DCM - RT.lvclass">, error out=w343:errorcluster, "Accessor:Setup:System"=w358:T8, "Accessor:Setup:PB"=w357:T8)
                              n168 = Strip Path(path=w353) -> (stripped path=w345:path)  [unwired: 1 out]
                              n169 = Strip Path(path=w345) -> (stripped path=w344:path)  [unwired: 1 out]
                              n170 = Unbundle By Name(w358) -> ("Model"=w361:u16, "Rev Major"=w342:u8)
                              n171 = Unbundle By Name(w357) -> ("Model"=w360:u16)
                              n172 = call <vilib>:"Close DCM Reference.vi"("DCM - RT in"=w354) -> ()  [unwired: 11 in]
                              n173 = Build Path(base path=w344, name or relative path="Data") -> (appended path=w351:path)
                              n174 = case shown="2316" w361 {
                                tunnel: w360 -> [_ _ _]
                                tunnel: [Bitfile_Selection."Unknown (Disabled)" ("DCM Model") w366 w379] -> w359
                                tunnel: [_ w365 w378] -> w347
                                tunnel: w351 -> [_ w364 w377]
                                tunnel: w342 -> [_ w363 w376]
                                frame Default {
                                }
                                frame 2301 {
                                n175 = case shown="4" w363 {
                                tunnel: [Bitfile_Selection."Unknown (Disabled)" ("DCM Model") Bitfile_Selection."DCM-2301" ("DCM Model") Bitfile_Selection."DCM-2301" ("DCM Model")] -> w366
                                tunnel: [_ w370 w374] -> w365
                                tunnel: w364 -> [_ w369 w373]
                                frame Default {
                                }
                                frame 4 {
                                n176 = Build Path(base path=w369, name or relative path="DCM - FPGA - 2316 - RevD.lvbitx") -> (appended path=w370:path)
                                }
                                frame 5 {
                                n177 = Build Path(base path=w373, name or relative path="DCM - FPGA - 2316 - RevE.lvbitx") -> (appended path=w374:path)
                                }
                                }
                                }
                                frame 2316 {
                                n178 = case shown="4" w376 {
                                tunnel: [Bitfile_Selection."Unknown (Disabled)" ("DCM Model") Bitfile_Selection."DCM-2316" ("DCM Model") Bitfile_Selection."DCM-2316" ("DCM Model")] -> w379
                                tunnel: [_ w383 w387] -> w378
                                tunnel: w377 -> [_ w382 w386]
                                frame Default {
                                }
                                frame 4 {
                                n179 = Build Path(base path=w382, name or relative path="DCM - FPGA - 2316 - RevD.lvbitx") -> (appended path=w383:path)
                                }
                                frame 5 {
                                n180 = Build Path(base path=w386, name or relative path="DCM - FPGA - 2316 - RevE.lvbitx") -> (appended path=w387:path)
                                }
                                }
                                }
                              }
                              n181 = Empty String/Path?(string/path=w348) -> (empty?=w350:bool)
                              n182 = Not(x=w350) -> (.not. x?=w349:bool)
                              n183 = Select(t=w348, s=w349, f=w347) -> (s? t:f=→"Local File Path":path)
                              n184 = property on="DCM Model" class="Enum (strict)"("Val(Sgnl)"=w359) -> ()  [unwired: 2 in, 2 out]
                            }
                            frame Error {
                              n185 = call <vilib>:"Close DCM Reference.vi"("DCM - RT in"=w390) -> ()  [unwired: 11 in]
                            }
                          }
                          n186 = local write "Status"("Reading Target" ("Status")) -> ()
                        }
                        frame 2, Default {
                          n187 = call <vilib>:"Unset Busy.vi"("error in (no error)"=w392, "VI reference (current VI)"=w394) -> ("error out"=w393:errorcluster)  [unwired: 9 in]
                          n188 = Close Reference(reference=w394, error in (no error)=w393) -> (error out=w391:errorcluster)
                          n189 = local write "Status"("Complete" ("Status")) -> ()
                        }
                      }
                    }
                    frame Error {
                      n190 = Close Reference(reference=w396) -> ()  [unwired: 1 in, 1 out]
                      n191 = local write "Status"("Error" ("Status")) -> ()
                    }
                  }
                }
              }
              frame True {
              }
            }
          }
          event "Clear": Mouse Down {
            n192 = event-data() -> ()  [unwired: 2 out]
            n193 = property on="DCM Model" class="Enum (strict)"("Val(Sgnl)"=Bitfile_Selection."Unknown (Disabled)" ("DCM Model")) -> ()  [unwired: 2 in, 2 out]
          }
        }
        n194 = call <vilib>:"Simple Error Handler.vi"("error in (no error)"=w120) -> ("error out"=w119:errorcluster)  [unwired: 1 in, 7 out]
        n195 = call <vilib>:"Clear Errors.vi"("error in (no error)"=w119) -> ("error out"=w118:errorcluster)  [unwired: 1 in, 5 out]
      }
      n196 = Unregister For Events(event registration refnum=w115, error in=w114) -> (error out=w113:errorcluster)
    }
    frame Error {
      n197 = call <vilib>:"Simple Error Handler.vi"("error in (no error)"=w403) -> ("error out"=w402:errorcluster)  [unwired: 1 in, 7 out]
      n198 = call <vilib>:"Clear Errors.vi"("error in (no error)"=w402) -> ("error out"=w401:errorcluster)  [unwired: 1 in, 5 out]
    }
  }
  n199 = invoke class="VI" method="FP.Close"(error in=w7) -> (error out=w6:errorcluster)  [unwired: 2 in, 2 out]
  n200 = call <vilib>:"NI VeriStand - Signal When Ready for Shutdown.vi"("error in (no error)"=w6) -> ("error out"=→"error out":errorcluster)  [unwired: 10 out]
